vi "Create Bulk CSV String.vi"(4 "Time Stamp Format":string="%Y%m%dT%H%M%S%3u", 6 "Delimiter":string=",", 8 "Error In":errorcluster, 10 "Messages":T1[](array[typedef]), 11 "Bulk CSV Buffer In":string) -> (0 "Error Out":errorcluster, 2 "CSV Length":i32, 3 "Bulk CSV Buffer Out":string)   [LabVIEW 2025, in "LOGlib_LV2025.lvlib" / "File.lvlib"]
uses:
  File.lvlib
  Type Definitions/Statement.ctl
  Type Definitions/Tag.ctl
  <vilib>/Utility/error.llb/Trim Whitespace.vi
  <vilib>/dlg_ctls.llb/Space Constant.vi
  <vilib>/Utility/error.llb/Trim Whitespace One-Sided.vi
  LOGlib_LV2025.lvlib
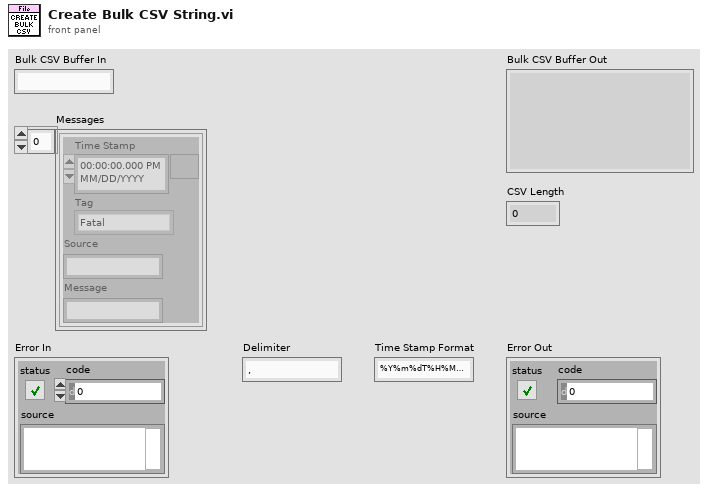
[diagram p1: front panel]
types:
  T1 = typedef "LOGlib_LV2025.lvlib/Statement.ctl" = cluster{"Time Stamp":timestamp, "Tag":T2, "Source":string, "Message":string}
  T2 = typedef "LOGlib_LV2025.lvlib/Tag.ctl" = enum16{"Fatal", "Error", "Warn", "Info", "Debug", "Trace"}
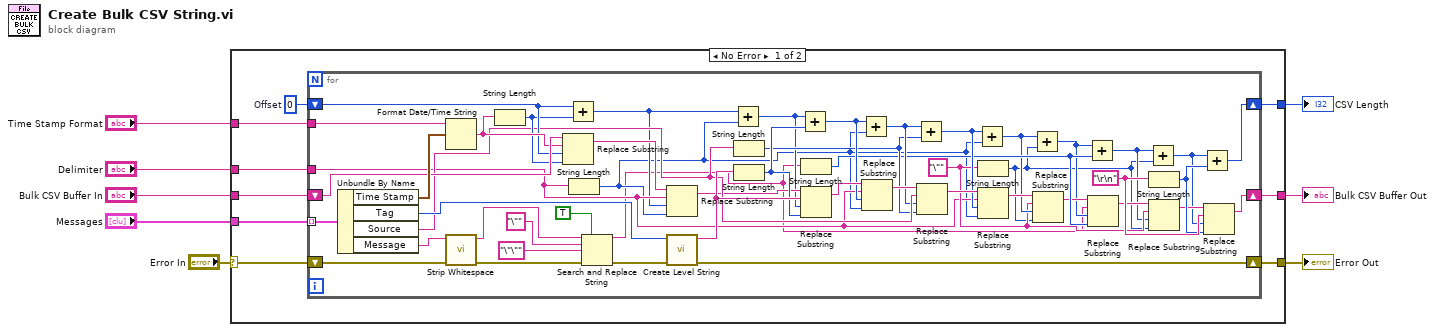
[diagram p0: block diagram]
diagram:
  n1 = case shown="No Error" "Error In" {
    selector: "Error In" -> [w17 w67]
    tunnel: [w16 w67] -> w7
    tunnel: "Messages" -> [w15 _]
    tunnel: "Bulk CSV Buffer In" -> [w14 _]
    tunnel: [w12 _] -> w4
    tunnel: [w11 _] -> w3
    tunnel: "Delimiter" -> [w10 _]
    tunnel: "Time Stamp Format" -> [w9 _]
    frame No Error {
      w13 = 0  # Offset
      n2 = for {
        tunnel: w15 -> [w66] mode=indexing
        shift-right: [w43] -> w12
        shift-left: w14 -> [w60]
        shift-right: [w62] -> w16
        shift-left: w17 -> [w64]
        shift-right: [w42] -> w11
        shift-left: w13 -> [w58]
        tunnel: w10 -> [w31]
        tunnel: w9 -> [w25]
        w35 = "\""
        w45 = "\r\n"
        n3 = Unbundle By Name(w66) -> ("Time Stamp"=w61:timestamp, "Tag"=w63:T2, "Source"=w51:string, "Message"=w65:string)
        n4 = Format Date/Time String(time format string (%c)=w25, seconds (now)=w61) -> (date/time string=w59:string)  [unwired: 1 in]
        n5 = call "Strip Whitespace.vi"("Error In"=w64, "Text"=w65) -> ("Error Out"=w24:errorcluster, "Stripped Text"=w21:string)  [unwired: 8 in]
        n6 = String Length(string=w59) -> (length=w57:i32)
        n7 = Replace Substring(2:w57, 3:w58, 4:w59, 5:w60) -> (1:w30:string)  [unwired: 1 out]
        n8 = Add(x=w58, y=w57) -> (x+y=w28:i32)
        n9 = String Length(string=w31) -> (length=w26:i32)
        n10 = Search and Replace String(replace all?=TRUE ("replace all? (F)"), input string=w21, search string="\"", replace string="\"\"" ("replace string (\"\")"), error in=w24) -> (result string=w20:string, error out=w23:errorcluster)  [unwired: 3 in, 2 out]
        n11 = Replace Substring(2:w26, 3:w28, 4:w31, 5:w30) -> (1:w29:string)  [unwired: 1 out]
        n12 = call "Create Level String.vi"("Error In"=w23, "Level"=w63) -> ("Error Out"=w62:errorcluster, "String"=w56:string)  [unwired: 8 in]
        n13 = Add(x=w28, y=w26) -> (x+y=w27:i32)
        n14 = String Length(string=w51) -> (length=w49:i32)
        n15 = String Length(string=w56) -> (length=w55:i32)
        n16 = Add(x=w27, y=w55) -> (x+y=w53:i32)
        n17 = String Length(string=w20) -> (length=w46:i32)
        n18 = Replace Substring(2:w55, 3:w27, 4:w56, 5:w29) -> (1:w54:string)  [unwired: 1 out]
        n19 = Add(x=w53, y=w26) -> (x+y=w50:i32)
        n20 = Replace Substring(2:w26, 3:w53, 4:w31, 5:w54) -> (1:w52:string)  [unwired: 1 out]
        n21 = Add(x=w50, y=w49) -> (x+y=w47:i32)
        n22 = Replace Substring(2:w49, 3:w50, 4:w51, 5:w52) -> (1:w48:string)  [unwired: 1 out]
        n23 = Add(x=w47, y=w26) -> (x+y=w39:i32)
        n24 = String Length(string=w35) -> (length=w33:i32)
        n25 = Replace Substring(2:w26, 3:w47, 4:w31, 5:w48) -> (1:w41:string)  [unwired: 1 out]
        n26 = Add(x=w39, y=w33) -> (x+y=w38:i32)
        n27 = Replace Substring(2:w33, 3:w39, 4:w35, 5:w41) -> (1:w40:string)  [unwired: 1 out]
        n28 = Add(x=w38, y=w46) -> (x+y=w34:i32)
        n29 = Replace Substring(2:w46, 3:w38, 4:w20, 5:w40) -> (1:w37:string)  [unwired: 1 out]
        n30 = Add(x=w34, y=w33) -> (x+y=w32:i32)
        n31 = String Length(string=w45) -> (length=w44:i32)
        n32 = Replace Substring(2:w33, 3:w34, 4:w35, 5:w37) -> (1:w36:string)  [unwired: 1 out]
        n33 = Add(x=w32, y=w44) -> (x+y=w42:i32)
        n34 = Replace Substring(2:w44, 3:w32, 4:w45, 5:w36) -> (1:w43:string)  [unwired: 1 out]
      }
    }
    frame Error {
    }
  }
  "Error Out" <- w7
  "Bulk CSV Buffer Out" <- w4
  "CSV Length" <- w3
